vi "GA Set Do Bit Reverse.vi"(7 "reverseTime":i16, 8 "error in (no error)":errorcluster caption="错误输入（无错误）", 9 "value":i32, 10 "nDoNum":i16, 11 "nDoType":i16) -> (0 "error out":errorcluster caption="错误输出", 3 "function return":i32)   [LabVIEW 2015, in "GAS.lvlib"]
doc: "extern \"C\" __declspec(dllimport) int GA_SetDoBitReverse(short nDoType,short nDoNum,long value,short reverseTime);"
uses:
  <userlib>/BP_GAS/GAS.lvlib
  <userlib>/BP_GAS/GAS.dll
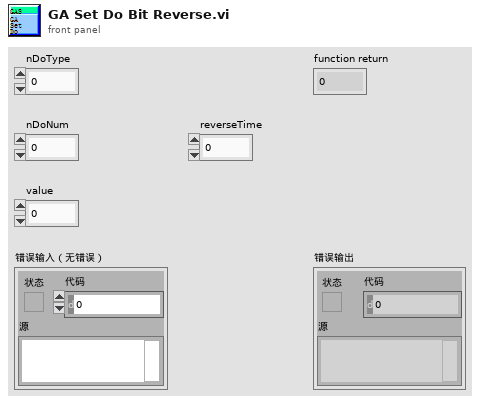
[diagram p1: front panel]
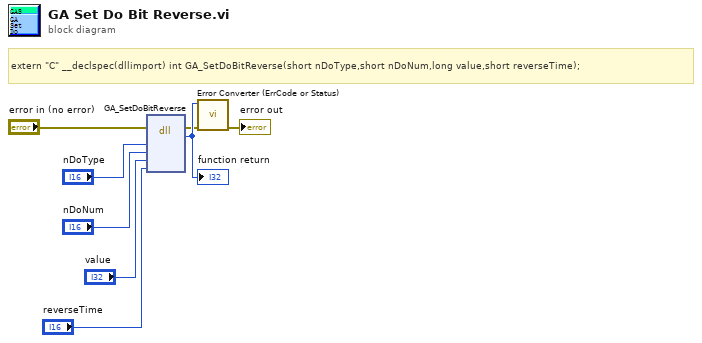
[diagram p0: block diagram]
diagram:
  # "extern \"C\" __declspec(dllimport) int GA_SetDoBitReverse(short nDoType,short nDoNum,long value,short reverseTime);"
  n1 = dll-call lib="E:/Program Files (x86)/National Instruments/LabVIEW 2015/user.lib/BP_GAS/GAS.*" fn="GA_SetDoBitReverse"(error in="error in (no error)", "nDoType"="nDoType", "nDoNum"="nDoNum", "value"="value", "reverseTime"="reverseTime") -> (error out=w2:errorcluster, w8:i32)  [unwired: 6 in, 1 out]
  "function return" <- w8
  n2 = call "Error Converter (ErrCode or Status).vi"("error in (no error)"=w2, "error code"=w8) -> ("error out"=→"error out":errorcluster)  [unwired: 9 in]
